vi "Compress Chunk.vi"(9 "Key Array":u32[](array[numeric]), 10 "Hash In":u32[](array[numeric]), 11 "Data Array In":u32[](array[numeric])) -> (3 "Hash Out":u32[](array[numeric]))   [LabVIEW 2019, in "SHA256.lvlib"]
doc: "Compresses chunks into the hash value.\n\nAfter the data to be encrypted has first been chunked into blocks of 16 x 32bit words, each chunk is extended over 64 x 32 bit words and then compressed, mixing in with a key and collected into a hash. This subvi does the compressing the extended chunks into the hash."
uses:
  Downloads/LabVIEW-Bits-master-2/Cryptographic Services/SHA256/SHA256.lvlib
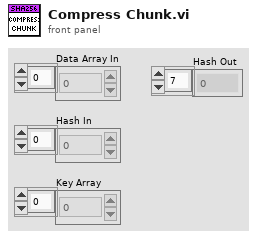
[diagram p1: front panel]
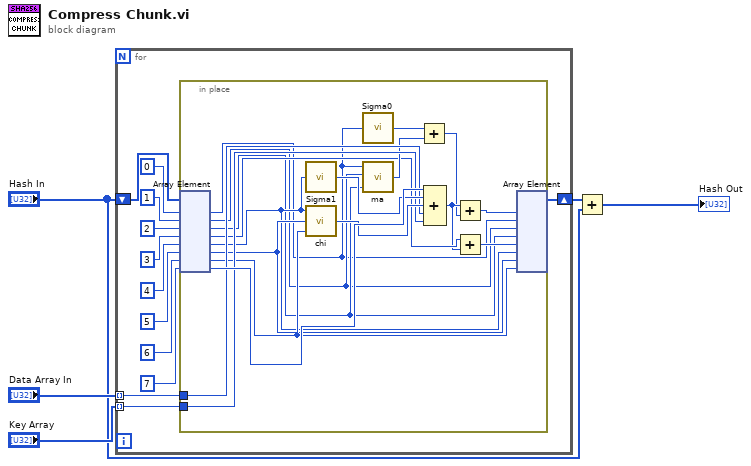
[diagram p0: block diagram]
diagram:
  n1 = for {
    tunnel: "Data Array In" -> [w8] mode=indexing
    tunnel: "Key Array" -> [w7] mode=indexing
    shift-right: [w6] -> w2
    shift-left: "Hash In" -> [w17]
    n2 = in-place {
      in-place-border: w8 -> [w32]
      in-place-border: w7 -> [w31]
      n3 = in-place-array #1(w17, 0, 1, 2, 3, 4, 5, 6, 7) -> (w21:u32, w22:u32, w23:u32, w25:u32, w26:u32, w27:u32, w28:u32, w35:u32)
      n4 = call "Sigma1.vi"("e"=w26) -> ("S1"=w34:u32)
      n5 = call "chi.vi"("g"=w28, "f"=w27, "e"=w26) -> ("ch"=w33:u32)
      n6 = call "Sigma0.vi"("a"=w21) -> ("S0"=w30:u32)
      n7 = call "ma.vi"("c"=w23, "b"=w22, "a"=w21) -> ("ma"=w29:u32)
      n8 = Add(x=w30, y=w29) -> (x+y=w19:u32)
      n9 = Compound Arithmetic op=ADD(w35, w34, w33, w32, w31) -> (w20:u32)
      n10 = Add(x=w20, y=w19) -> (x+y=w18:u32)
      n11 = Add(x=w25, y=w20) -> (x+y=w24:u32)
      n12 = in-place-array #1(w18, w21, w22, w23, w24, w26, w27, w28) -> (w6:u32[])  [unwired: 8 out]
    }
  }
  n13 = Add(x=w2, y="Hash In") -> (x+y=→"Hash Out":u32[])
